vi "ExitWindowsEx.vi"(8 "error in (no error)":errorcluster, 10 "force function (0 - No force)":i32(ring) items=["No force", "Force", "Force if Hung"], 11 "exit function (0 - Logoff)":i32(ring) items=["Logoff", "Shutdown System", "Reboot System", "Poweroff System"]) -> (0 "error out":errorcluster)   [LabVIEW 2011]
doc: "ExitWindowsEx\nThe ExitWindowsEx function either logs off the current user, shuts down the system, or shuts down and restarts the system. It sends the WM_QUERYENDSESSION message to all applications to determine if they can be terminated. \n\nBOOL ExitWindowsEx(\n UINT uFlags, // shutdown operation\n DWORD dwReserved // reserved\n);\n \nParameters\nuFlags \nSpecifies the type of shutdown. This parameter must include one of the following values: Value Meaning \nEWX_LOGOFF Shuts down all processes running in the security context of the process that called the ExitWindowsEx function. Then it logs the user off. \nEWX_POWEROFF Shuts down the system and turns off the power. The system must support the power-off feature.\nWindows NT: The calling process must have the SE_SHUTDOWN_NAME privilege. For more information, see the following Remarks section. \n \nEWX_REBOOT Shuts down the system and then restarts the system. \nWindows NT: The calling process must have the SE_SHUTDOWN_NAME privilege. For more information, see the following Remarks section. \n \nEWX_SHUTDOWN Shuts down the system to a point at which it is safe to turn off the power. All file buffers have been flushed to disk, and all running processes have stopped. \nWindows NT: The calling process must have the SE_SHUTDOWN_NAME privilege. For more information, see the following Remarks section. \n \n\n\nThis parameter can optionally include the following values: Value Meaning \nEWX_FORCE Forces processes to terminate. When this flag is set, the system does not send the WM_QUERYENDSESSION and WM_ENDSESSION messages. This can cause the applications to lose data. Therefore, you should only use this flag in an emergency. \nEWX_FORCEIFHUNG Windows NT 5.0 and later: Forces processes to terminate if they do not respond to the WM_QUERYENDSESSION or WM_ENDSESSION message. This flag is ignored if EWX_FORCE is used. \n\n\n\ndwReserved \nReserved; this parameter is ignored. \nReturn Values\nIf the function succeeds, the return value is nonzero.\n\nIf the function fails, the return value is zero. To get extended error information, callGetLastError. \n\nRemarks\nThe ExitWindowsEx function returns as soon as it has initiated the shutdown. The shutdown or logoff then proceeds asynchronously. \n\nDuring a shutdown or log-off operation, applications that are shut down are allowed a specific amount of time to respond to the shutdown request. If the time expires, the system displays a dialog box that allows the user to forcibly shut down the application, to retry the shutdown, or to cancel the shutdown request. If the EWX_FORCE value is specified, the system always forces applications to close and does not display the dialog box. If the EWX_FORCEIFHUNG value is specified, the system forces hung applications to close and does not display the dialog box. \n\nConsole processes receive a separate notification message, CTRL_SHUTDOWN_EVENT or CTRL_LOGOFF_EVENT, as the situation warrants. A console process routes these messages to its HandlerRoutine functions, which are added and removed by calls to the SetConsoleCtrlHandler function. ExitWindowsEx sends these notification messages asynchronously; thus, an application cannot assume that the console notification messages have been handled when a call to ExitWindowsEx returns. \n\nWindows NT: To shut down or restart the system, the calling process must use theAdjustTokenPrivileges function to enable the SE_SHUTDOWN_NAME privilege. For more information about security privileges, seePrivileges. \n\nWindows 95: ExitWindowEx does not work from a console application, as it does on Windows NT."
uses:
  user32.dll
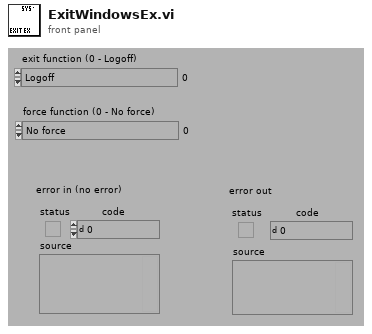
[diagram p1: front panel]
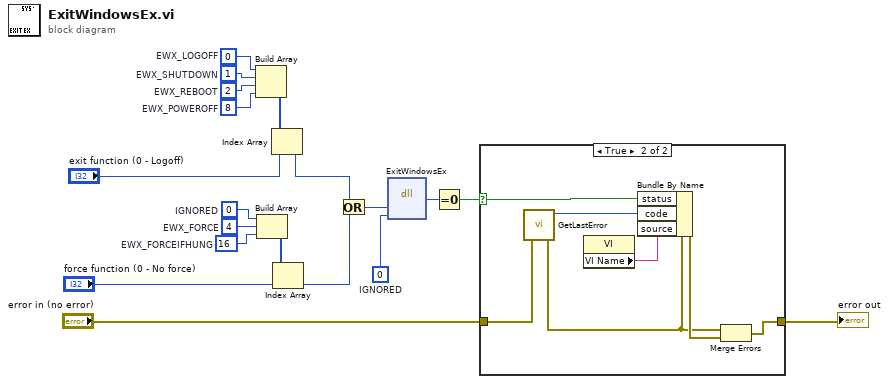
[diagram p0: block diagram]
diagram:
  w5 = u16 0  # IGNORED
  w12 = u32 0  # IGNORED
  w10 = u32 16  # EWX_FORCEIFHUNG
  w11 = u32 4  # EWX_FORCE
  w19 = u32 1  # EWX_SHUTDOWN
  w18 = u32 0  # EWX_LOGOFF
  w16 = u32 8  # EWX_POWEROFF
  w17 = u32 2  # EWX_REBOOT
  n1 = Build Array(w18, w19, w17, w16) -> (w15:u32[])
  n2 = Build Array(w12, w11, w10) -> (w9:u32[])
  n3 = Index Array(array=w15, index="exit function (0 - Logoff)") -> (element=w14:u32)
  n4 = Index Array(array=w9, index="force function (0 - No force)") -> (element=w8:u32)
  n5 = Or(x=w14, y=w8) -> (x .or. y?=w13:u32)
  n6 = dll-call lib="User32.dll" fn="ExitWindowsEx"("uFlags"=w13, "reserved (set to zero)"=w5) -> (w6:i16)  [unwired: 5 in, 2 out]
  n7 = Equal To 0?(x=w6) -> (x = 0?=w3:bool)
  n8 = case shown="True" w3 {
    selector: w3 -> [_ w25]
    tunnel: [w20 w23] -> w1
    tunnel: "error in (no error)" -> [w20 w22]
    frame False {
    }
    frame True {
      n9 = call "GetLastError.vi"("error in (no error)"=w22) -> ("error out"=w21:errorcluster, "CODE"=w27:i32)  [unwired: 5 out]
      n10 = property class="VI"() -> ("VI Name"=w26:string)  [unwired: 2 in, 2 out]
      n11 = Bundle By Name(cluster=w21, "status"=w25, "code"=w27, "source"=w26) -> (w24:errorcluster)
      n12 = Merge Errors(w21, w24) -> (w23:errorcluster)
    }
  }
  "error out" <- w1
